vi "FSM.vi"(3 "Init State":T1=enum."Plus") -> (1 "Current\nState":T1)   [LabVIEW 2017]
uses:
  States.ctl
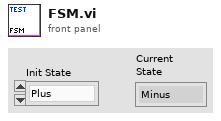
[diagram p1: front panel]
types:
  T1 = typedef "States.ctl" = enum16{"Minus", "Zero", "Plus"}
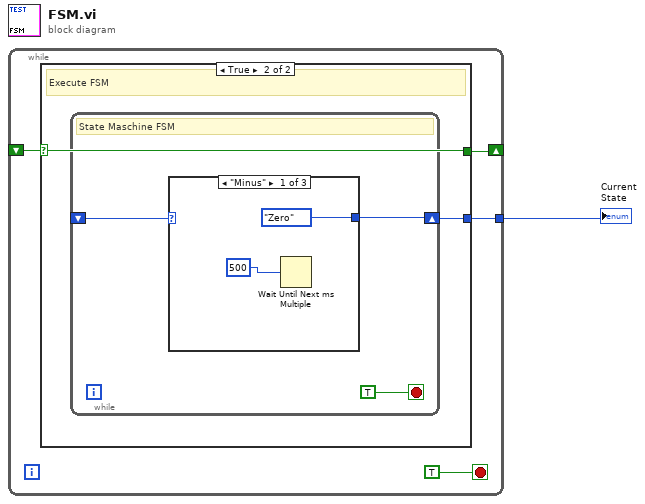
[diagram p0: block diagram]
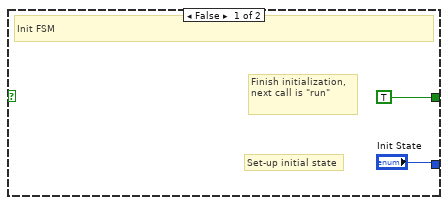
[diagram p2: hidden frame]
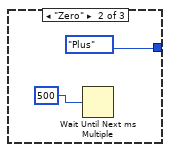
[diagram p3: hidden frame]
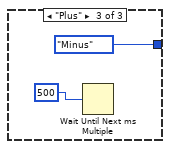
[diagram p4: hidden frame]
diagram:
  n1 = while {
    tunnel: [w5] -> w1
    shift-right: [w2] -> _
    shift-left: _ -> [w3]
    stop <- TRUE stop-if-true
    n2 = case shown="True" w3 {
      selector: w3 -> [_ w8]
      tunnel: ["Init State" w9] -> w5
      tunnel: [TRUE w8] -> w2
      frame False {
        # "Finish initialization, \nnext call is \"run\""
        # "Set-up initial state"
        # "Init FSM"
      }
      frame True {
        # "Execute FSM"
        n3 = while {
          shift-right: [w12] -> w9
          shift-left: _ -> [w10]
          stop <- TRUE stop-if-true
          # "State Maschine FSM"
          n4 = case shown="\"Minus\"" w10 {
            tunnel: [States."Zero" ("State") States."Plus" ("State 2") States."Minus" ("State")] -> w12
            frame "Minus" {
              n5 = Wait Until Next ms Multiple(millisecond multiple=500) -> ()  [unwired: 1 out]
            }
            frame "Zero" {
              n6 = Wait Until Next ms Multiple(millisecond multiple=500) -> ()  [unwired: 1 out]
            }
            frame "Plus" {
              n7 = Wait Until Next ms Multiple(millisecond multiple=500) -> ()  [unwired: 1 out]
            }
          }
        }
      }
    }
  }
  "Current\nState" <- w1
